vi "Resolve New State.vi"(8 "error in":errorcluster, 10 "Received Test Event":T1, 11 "Current State":T2) -> (0 "error out":errorcluster, 3 "New State":T2)   [LabVIEW 2009, in "Caraya.lvlib" / "Basic Test Manager.lvclass"]
uses:
  Basic Test Manager.lvclass
  Test State.ctl
  Assert Event Data.ctl
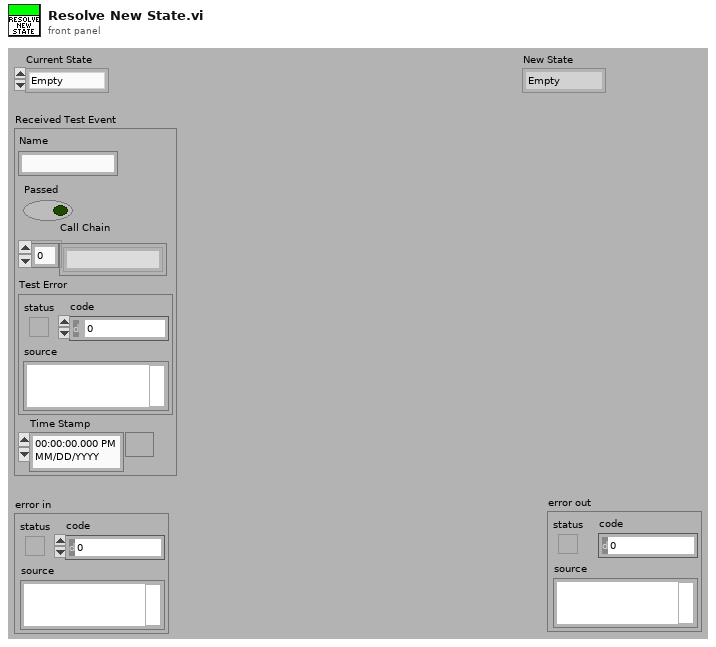
[diagram p1: front panel]
types:
  T1 = typedef "Caraya.lvlib/Basic Test Manager.lvclass/Assert Event Data.ctl" = cluster{"Name":string, "Passed":bool, "Call Chain":string[], "Test Error":errorcluster, "Time Stamp":timestamp}
  T2 = typedef "Caraya.lvlib/Basic Test Manager.lvclass/Test State.ctl" = enum16{"Empty", "Unknown", "Fail", "Pass", "Skip", "Error"}
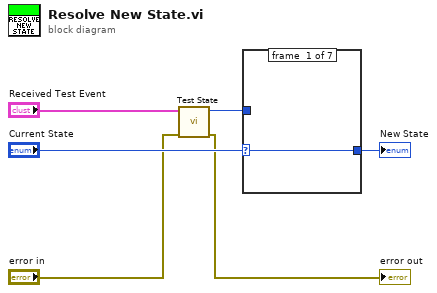
[diagram p0: block diagram]
diagram:
  n1 = call "Test State.vi"("error in (no error)"="error in", "Test Event"="Received Test Event") -> ("error out"=→"error out":errorcluster, "Test State"=w5:T2)  [unwired: 8 in]
  n2 = case shown="\"Error\"" "Current State" {
    selector: "Current State" -> [w7 _ w9 _ w12 w17 _]
    tunnel: w5 -> [_ w8 _ w10 w13 w18 w21]
    tunnel: [w7 w8 w9 w10 w11 w16 w21] -> w6
    frame #0 {
    }
    frame #1 {
    }
    frame #2 {
    }
    frame #3 {
    }
    frame #4 {
      n3 = case shown="\"Fail\"" w13 {
        selector: w13 -> [_ w15]
        tunnel: w12 -> [w14 _]
        tunnel: [w14 w15] -> w11
        frame #0 {
        }
        frame #1 {
        }
      }
    }
    frame #5 {
      n4 = case shown="Default" w18 {
        selector: w18 -> [_ w20]
        tunnel: w17 -> [w19 _]
        tunnel: [w19 w20] -> w16
        frame #0 {
        }
        frame #1 {
        }
      }
    }
    frame #6 {
    }
  }
  "New State" <- w6
